vi "SortinData.vi"(3 "binning":dbl format="%.2f", 4 "Array sop":u32[][](array[numeric]), 8 "rawdata":T1, 9 "MAT trace/retrace":dbl format="%.2f") -> (11 "trace photons":i32, 14 "valid":i32, 16 "invalid":i32, 17 "gap":i32, 19 "Array sop 2":u32[][](array[numeric]))   [LabVIEW 2009]
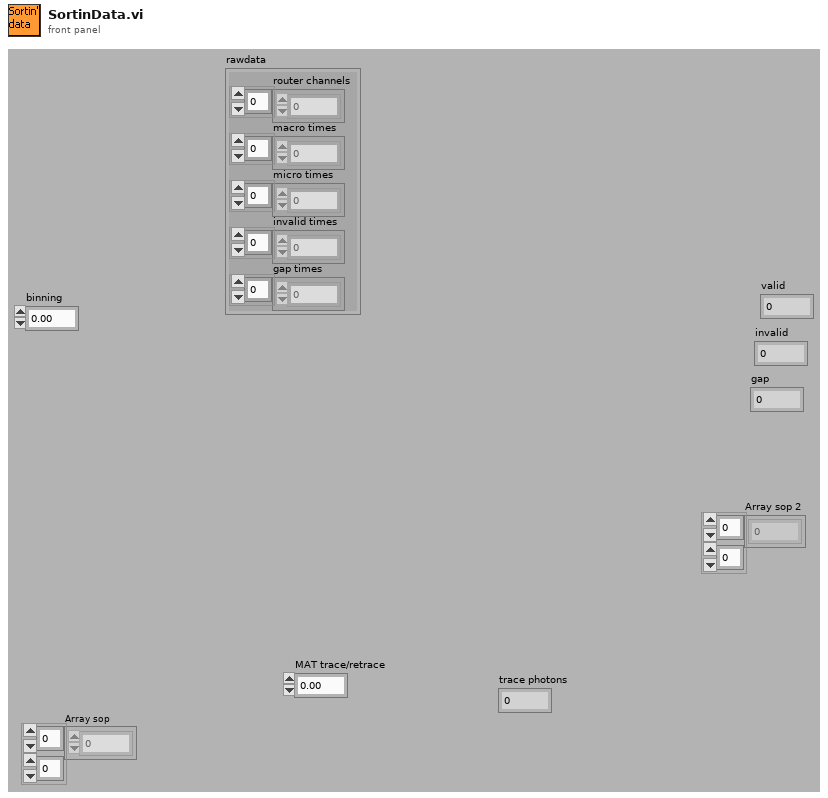
[diagram p1: front panel]
types:
  T1 = cluster{"router channels":u8[], "macro times":dbl[], "micro times":u16[], "invalid times":dbl[], "gap times":dbl[]}
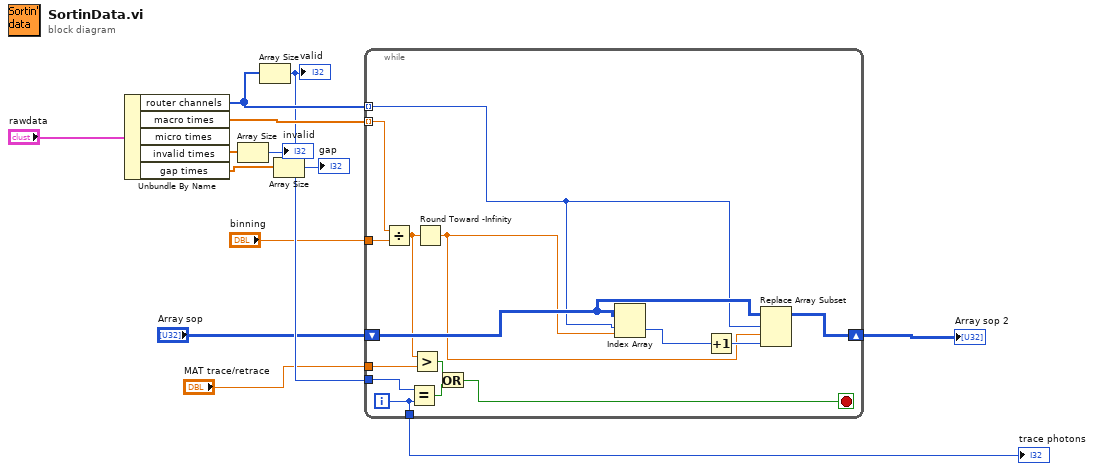
[diagram p0: block diagram]
diagram:
  n1 = Unbundle By Name("rawdata") -> ("router channels"=w7:u8[], "macro times"=w12:dbl[], "invalid times"=w11:dbl[], "gap times"=w10:dbl[])  [unwired: 1 out]
  n2 = Array Size(array=w11) -> (size(s)=→"invalid":i32)
  n3 = Array Size(array=w7) -> (size(s)=w6:i32)
  "valid" <- w6
  n4 = Array Size(array=w10) -> (size(s)=→"gap":i32)
  n5 = while {
    tunnel: w7 -> [w16] mode=indexing
    tunnel: w12 -> [w19] mode=indexing
    tunnel: "binning" -> [w28]
    shift-right: [w25] -> w2
    shift-left: "Array sop" -> [w26]
    tunnel: w6 -> [w24]
    tunnel: "MAT trace/retrace" -> [w23]
    tunnel: [w17] -> w4
    i -> [w17]
    stop <- w20 stop-if-true
    n6 = Divide(x=w19, y=w28) -> (x/y=w18:dbl)
    n7 = Equal?(x=w24, y=w17) -> (x = y?=w21:bool)
    n8 = Greater?(x=w18, y=w23) -> (0:w22:bool)
    n9 = Round Toward -Infinity(1:w18) -> (0:w14:dbl)
    n10 = Or(x=w22, y=w21) -> (x .or. y?=w20:bool)
    n11 = Index Array(array=w26, index (row)=w16, index (col)=w14) -> (element=w15:u32)
    n12 = Increment(x=w15) -> (x+1=w27:u32)
    n13 = Replace Array Subset(array=w26, new element=w27, index (row)=w16, index (col)=w14) -> (w25:u32[][])
  }
  "trace photons" <- w4
  "Array sop 2" <- w2
